vi "Set Analysis Z ROI.vi"(8 "error in (no error)":errorcluster, 11 "Analysis Graph in":refnum<class "Analysis Graph.lvclass">) -> (0 "error out":errorcluster, 3 "Analysis Graph out":refnum<class "Analysis Graph.lvclass">)   [LabVIEW 2023, in "Analysis Graph.lvclass"]
uses:
  Analysis Graph.lvclass
  Analysis Graph.lvclass/Analysis Graph.ctl
panel:
  in  "Z Range":cluster{"Index":u32, "Length":u32}
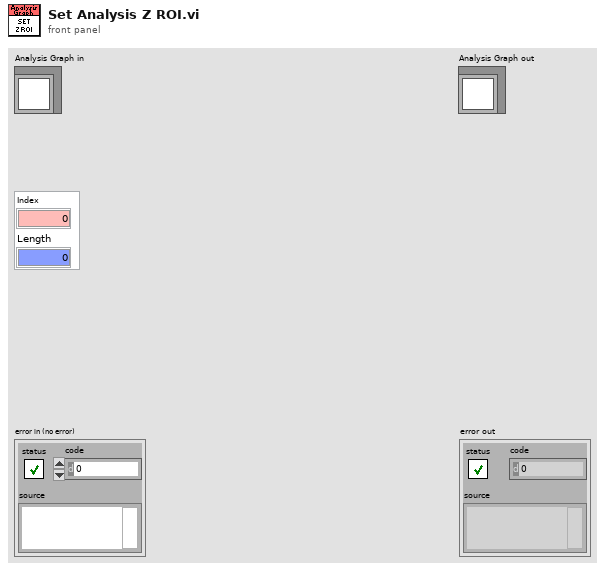
[diagram p1: front panel]
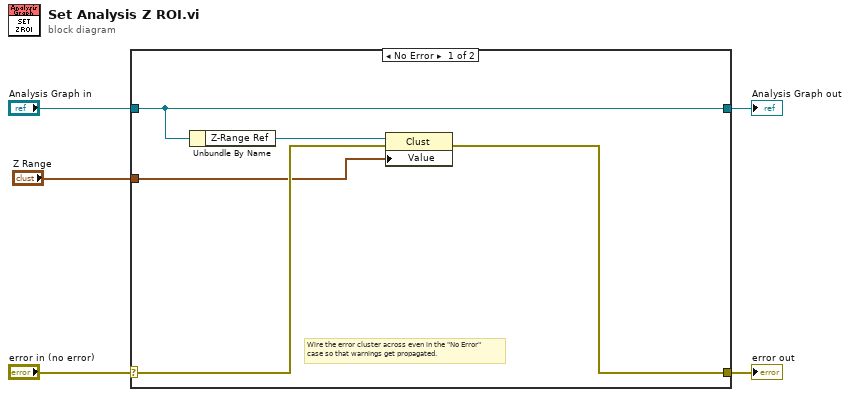
[diagram p0: block diagram]
diagram:
  n1 = case shown="No Error" "error in (no error)" {
    selector: "error in (no error)" -> [w9 w12]
    tunnel: [w7 w12] -> w4
    tunnel: [w6 w11] -> w2
    tunnel: "Analysis Graph in" -> [w6 w11]
    tunnel: "Z Range" -> [w8 _]
    frame No Error {
      # "Wire the error cluster across even in the \"No Error\"\ncase so that warnings get propagated."
      n2 = Unbundle By Name(w6) -> ("Z-Range Ref"=w10:refnum<vi>)
      n3 = property class="Clust"(reference=w10, error in=w9, "Value"=w8) -> (error out=w7:errorcluster)  [unwired: 1 out]
    }
    frame Error {
    }
  }
  "error out" <- w4
  "Analysis Graph out" <- w2
